vi "Create.vi"(7 "Direction":T1, 8 "error in (no error)":errorcluster, 9 "Custom Config Data":u8[](array[numeric]), 10 "Name":string, 11 "CIFTag in":refnum<class "CIF_CIPC_Chn_String.lvclass">) -> (0 "error out":errorcluster, 3 "CIFTag out":refnum<class "CIF_CIPC_Chn_String.lvclass">)   [LabVIEW 2021, in "CIF_CIPC_Chn_String.lvclass"]
uses:
  CIF_CIPC_Chn_String.lvclass
  D:/dev/Packages/CIF_Channels_Core/src/CIFChannels/CIFChannels.lvclass
  D:/dev/Packages/CIF_Channels_Core/src/CIPC_Channels/CIF_CIPC_Chan/CIF_CIPC_Chn.lvclass
  ChannelCommon/typedef/Direction.ctl
  <vilib>/Utility/Data Type/Type Definitions/Data Type.ctl
  ChannelCommon/typedef/Channel Pattern.ctl
  ChannelCommon/typedef/Disconnect Behavior.ctl
  CIF_CIPC_Chan/Typedef/Buffer Configuration Data.ctl
  <vilib>/CIF Foundation/CIF CIPC/TypeDefs/Backpressure References.ctl
  <vilib>/CIF Foundation/CIF CIPC/TypeDefs/Backpressure Names.ctl
  ChannelCommon/typedef/Channel State.ctl
  CIF_CIPC_Chan/CIF_CIPC_Chn.lvclass/CIF_CIPC_Chn.ctl
  CIF_CIPC_Chn_String.lvclass/CIF_CIPC_Chn_String.ctl
  CIFChannels/CIFChannels.lvclass/CIFChannels.ctl
  df6797b5-3f3a-463f-a676-d85c8ce06da0.vi
  3e71386b-e635-4616-ad06-93410a9d2207.vi
  CIF_CIPC_Chan/Accessors/Write CIPC Channel.vi
  CIF_CIPC_Chan/Accessors/Write Buffer Configuration.vi
  CIFChannels/Accessors/Write Channel State.vi
  CIFChannels/Accessors/Write Pattern.vi
  CIF_CIPC_Chan/Accessors/Write Data Type.vi
  df6797b5-3f3a-463f-a676-d85c8ce06da0.vi/bd07d5d9-1209-45ad-b636-9e9ab86132fb.vi
  <vilib>/CIF Foundation/CIF CIPC/SubVIs/Check Error.vi
  <vilib>/CIF Foundation/CIF CIPC/SubVIs/Add CIPC Error.vi
  <vilib>/CIF Foundation/CIF CIPC/SubVIs/Get dll Path.vi
  <vilib>/CIF Foundation/CIF CIPC/SubVIs/Notify Of New Write.vi
  <vilib>/CIF Foundation/CIF CIPC/SubVIs/Get Element Write Position.vi
  <vilib>/CIF Foundation/CIF CIPC/SubVIs/Get Element Description Variant.vi
  <vilib>/Utility/error.llb/Trim Whitespace.vi
  <vilib>/string/Create NI GUID.vi
  <vilib>/CIF Foundation/CIF CIPC/SubVIs/Check Error Core.vi
  <vilib>/CIF Foundation/CIF CIPC/SubVIs/Add CIPC Error Core.vi
  <vilib>/CIF Foundation/CIF CIPC/SubVIs/Get Element Info Variant.vi
  CIFChannels/CIFChannels.lvclass
  ChannelCommon/ChannelCommon.lvlib
  <vilib>/CIF Foundation/CIF CIPC/CIF_NI_CIPC.lvlib
  CIF_CIPC_Chan/CIF_CIPC_Chn.lvclass
  <vilib>/Utility/Data Type/NI_Data Type.lvlib
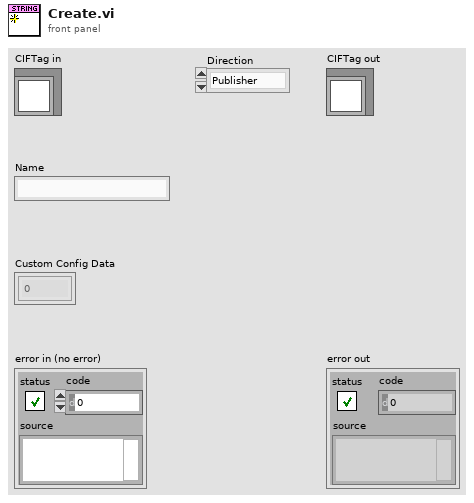
[diagram p1: front panel]
types:
  T1 = typedef "ChannelCommon.lvlib/Direction.ctl" = enum8{"Publisher", "Subscriber"}
  T2 = typedef "NI_Data Type.lvlib/Data Type.ctl" = enum8{"Invalid Type", "Void", "I8", "I16", "I32", "I64", "U8", "U16", "U32", "U64", "Single Float", "Double Float", "Extended Float", "Single Complex", "Double Complex", "Extended Complex", "Enum U8", "Enum U16", "Enum U32", "Enum U64", "Single Float With Unit", "Double Float With Unit", "Extended Float With Unit", "Single Complex with Unit", "Double Complex with Unit", "Extended Complex with Unit", "Boolean", "String", "Path", "Picture", "Tag", "Array", "Cluster", "Variant", "LV Variant", "Waveform", "Timestamp", "Digital Waveform", "Digital Data", "ExpressData", "Refnum", "External Data", "VI", "Poly VI", "LabVIEW Class Instance", "Fixed Point", "Set Collection", "Map Collection"}
  T3 = typedef "ChannelCommon.lvlib/Channel Pattern.ctl" = enum8{"Unknown", "Tag", "FIFO", "MultiFIFO", "BackpressureFIFO"}
  T4 = typedef "ChannelCommon.lvlib/Disconnect Behavior.ctl" = enum8{"Default value", "Last value", "Error with default"}
  T5 = typedef "CIF_CIPC_Chn.lvclass/Buffer Configuration Data.ctl" = cluster{"Total Size":u32, "Read Size":u32, "Read Offset":u32, "CIPC BP References":T6, "CIPC Backpressure Names":T7, "Override CIPC Name":string, "Encoder Data":string}
  T6 = typedef "CIF_NI_CIPC.lvlib/Backpressure References.ctl" = cluster{"CIPC Reference":u64, "CIPC BP Reference":u64}
  T7 = typedef "CIF_NI_CIPC.lvlib/Backpressure Names.ctl" = cluster{"CIPC Name":string, "CIPC BP Name":string}
  T8 = typedef "ChannelCommon.lvlib/Channel State.ctl" = enum8{"Creating", "Disconnected", "Connecting", "Connected", "Destroyed"}
  T9 = typedef "CIF_NI_CIPC.lvlib/Encoder Info.ctl" = cluster{"Name":string, "Version":i32, "Data":string}
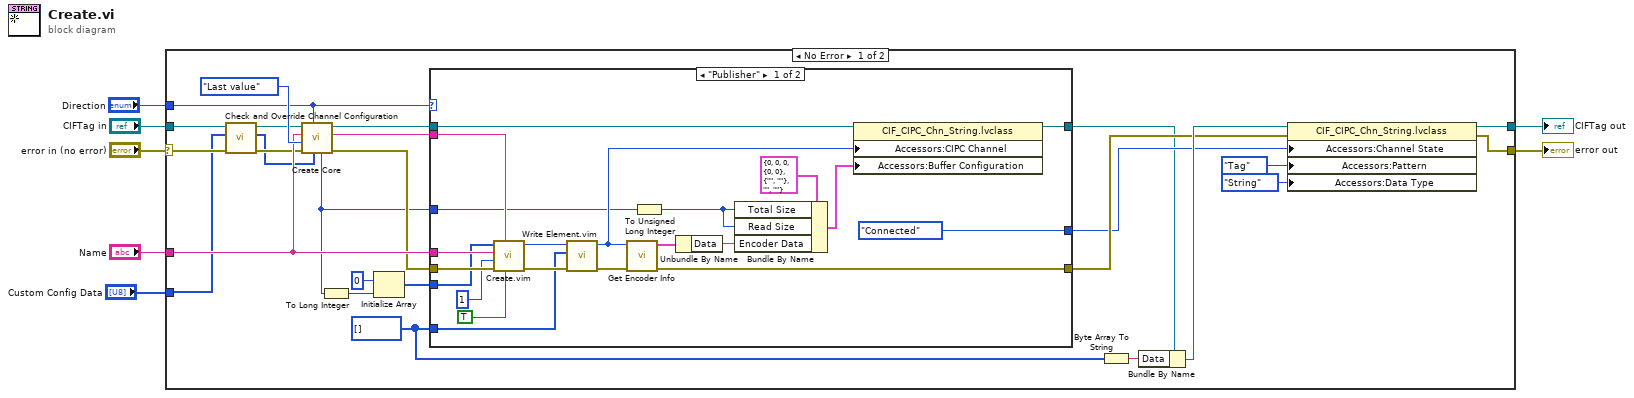
[diagram p0: block diagram]
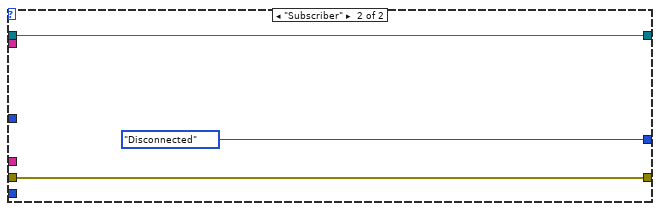
[diagram p2: hidden frame]
diagram:
  n1 = case shown="No Error" "error in (no error)" {
    selector: "error in (no error)" -> [w18 w59]
    tunnel: [w32 w59] -> w1
    tunnel: [w28 w58] -> w5
    tunnel: "CIFTag in" -> [w20 w58]
    tunnel: "Name" -> [w31 _]
    tunnel: "Direction" -> [w27 _]
    tunnel: "Custom Config Data" -> [w16 _]
    frame No Error {
      w10 = u8[] []
      n2 = call-dynamic "Check and Override Channel Configuration.vi"("error in (no error)"=w18, "Custom Config Data in"=w16, "CIF_CIPC_Chn_String in"=w20) -> ("error out"=w17:errorcluster, "Custom Config Data out"=w15:u8[], "CIF_CIPC_Chn_String out"=w19:refnum<class "CIF_CIPC_Chn_String.lvclass">)  [unwired: 6 in]
      n3 = call "Create Core.vi"("Custom Config Data"=w15, "Direction"=w27, "error in (no error)"=w17, "Disconnect Behavior"=Disconnect_Behavior."Last value", "Name"=w31, "CIFChannels in"=w19) -> ("error out"=w25:errorcluster, "Channel Type"=w23:string, "CIFChannels out"=w22:refnum<class "CIF_CIPC_Chn_String.lvclass">, "Bytes/Msg"=w9:u64)  [unwired: 1 in, 1 out]
      n4 = To Long Integer(number=w9) -> (32bit integer=w14:i32)
      n5 = Initialize Array(u8 0 ("Buffer Size N (2^N)"), w14) -> (w13:u8[])
      n6 = case shown="\"Publisher\"" w27 {
        tunnel: w31 -> [w50 _]
        tunnel: w25 -> [w51 w56]
        tunnel: w13 -> [w47 _]
        tunnel: [w39 w56] -> w29
        tunnel: [Channel_State."Connected" ("Channel State") Channel_State."Disconnected" ("Channel State")] -> w26
        tunnel: w23 -> [w48 _]
        tunnel: w22 -> [w46 w55]
        tunnel: [w38 w55] -> w21
        tunnel: w10 -> [w36 _]
        tunnel: w9 -> [w35 _]
        frame "Publisher" {
          n7 = call "Create.vim"("Prepend Array Size"=TRUE, "Description"=w48, "error in (no error)"=w51, "Buffer Size N (2^N)"=u8 1, "Name in"=w50, "Data Type"=w47) -> ("error out"=w52:errorcluster, "CIPC Reference"=w53:u64)  [unwired: 2 in, 2 out]
          n8 = call "Write Element.vim"("error in (no error)"=w52, "Data in"=w36, "CIPC Reference in"=w53) -> ("error out"=w45:errorcluster, "CIPC Reference out"=w44:u64)  [unwired: 5 in, 2 out]
          n9 = call <vilib>:"Get Encoder Info.vi"("error in (no error)"=w45, "CIPC Reference"=w44) -> ("error out"=w39:errorcluster, "Encoder Info"=w43:T9)  [unwired: 8 in]
          n10 = To Unsigned Long Integer(number=w35) -> (unsigned 32bit integer=w34:u32)
          n11 = Unbundle By Name(w43) -> ("Data"=w42:string)
          n12 = Bundle By Name(cluster=T5 {"Total Size"=0, "Read Size"=0, "Read Offset"=0, "CIPC BP References"={"CIPC Reference"=0, "CIPC BP Reference"=0}, "CIPC Backpressure Names"={"CIPC Name"="", "CIPC BP Name"=""}, "Override CIPC Name"="", "Encoder Data"=""} ("Buffer Configuration"), "Total Size"=w34, "Read Size"=w34, "Encoder Data"=w42) -> (w41:T5)
          n13 = property class="CIF_CIPC_Chn_String.lvclass"(reference=w46, "Accessors:CIPC Channel"=w44, "Accessors:Buffer Configuration"=w41) -> (reference out=w38:refnum<class "CIF_CIPC_Chn_String.lvclass">)  [unwired: 1 in, 1 out]
        }
        frame "Subscriber" {
        }
      }
      n14 = Byte Array To String(unsigned byte array=w10) -> (string=w11:string)
      n15 = Bundle By Name(cluster=w21, "Data"=w11) -> (w30:refnum<class "CIF_CIPC_Chn_String.lvclass">)
      n16 = property class="CIF_CIPC_Chn_String.lvclass"(reference=w30, error in=w29, "Accessors:Channel State"=w26, "Accessors:Pattern"=Channel_Pattern."Tag" ("Pattern"), "Accessors:Data Type"=Data_Type."String" ("Data Type")) -> (reference out=w28:refnum<class "CIF_CIPC_Chn_String.lvclass">, error out=w32:errorcluster)
    }
    frame Error {
    }
  }
  "error out" <- w1
  "CIFTag out" <- w5
